vi "__READ_PM_1ch_E4419A.VI"(7 "GPIB":string="13") -> (3 "chA":dbl=-19.9032016 format="%.4f")   [LabVIEW 2017]
panel:
  # "TPD//133.40.220.247//2"
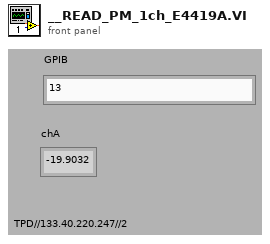
[diagram p1: front panel]
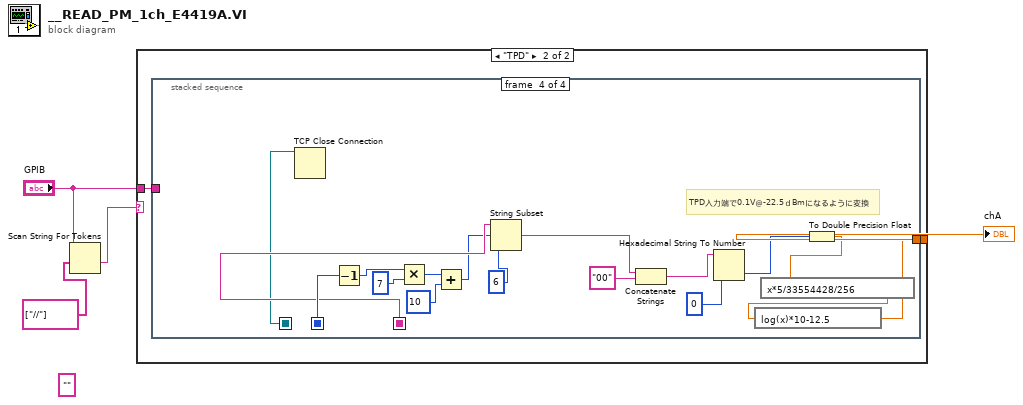
[diagram p0: block diagram]
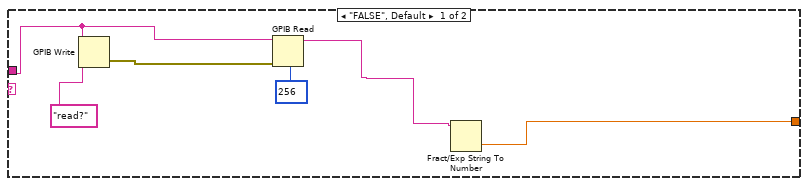
[diagram p2: hidden frame]
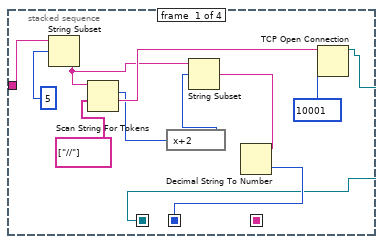
[diagram p3: hidden frame]
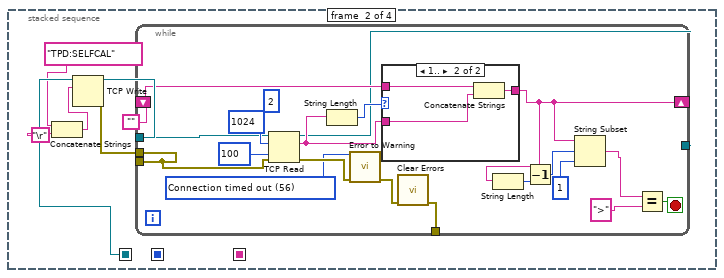
[diagram p4: hidden frame]
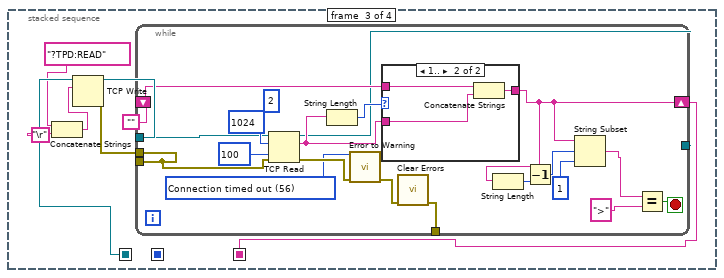
[diagram p6: hidden frame]
diagram:
  (unwired) ""
  n1 = Scan String For Tokens(7:string[] ["//"], 9:"GPIB") -> (1:w1:string)  [unwired: 4 in, 3 out]
  n2 = case shown="\"TPD\"" w1 {
    tunnel: [w10 w11] -> w4
    tunnel: "GPIB" -> [w5 w12]
    frame "FALSE", Default {
      n3 = GPIB Write(0:w5, 1:"read?") -> (6:w6:errorcluster)  [unwired: 3 in, 1 out]
      n4 = GPIB Read(0:w5, 1:256, 3:w6) -> (5:w9:string)  [unwired: 2 in, 2 out]
      n5 = Fract/Exp String To Number(string=w9) -> (number=w10:dbl)  [unwired: 3 in, 1 out]
    }
    frame "TPD" {
      n6 = stacked-sequence {
        seq-local: [w13 _ _ _] -> [_ w30 w61 w85]
        seq-local: [w14 _ _ _] -> [_ _ _ w101]
        seq-local: [_ _ w57 _] -> [_ _ _ w96]
        tunnel: w12 -> [w21 _ _ _]
        tunnel: [_ _ _ w86] -> w11
        frame #0 {
          n7 = String Subset(string=w21, offset (0)=5) -> (substring=w16:string)  [unwired: 1 in]
          n8 = Scan String For Tokens(7:string[] ["//"], 9:w16) -> (1:w20:string, 2:w19:i32)  [unwired: 4 in, 2 out]
          n9 = expression code="x+2"(w19) -> (w18:i32)
          n10 = String Subset(string=w16, offset (0)=w18) -> (substring=w17:string)  [unwired: 1 in]
          n11 = Decimal String To Number(string=w17) -> (number=w14:i32)  [unwired: 2 in, 1 out]
          n12 = TCP Open Connection(address=w20, remote port or service name=10001) -> (connection ID=w13:refnum<k5>)  [unwired: 3 in, 1 out]
        }
        frame #1 {
          n13 = Concatenate Strings("TPD:SELFCAL", "\r") -> (w24:string)
          n14 = TCP Write(connection ID=w30, data in=w24) -> (connection ID out=w28:refnum<k5>, error out=w27:errorcluster)  [unwired: 2 in, 1 out]
          n15 = while {
            tunnel: w28 -> [w48]
            shift-right: [w41] -> _
            shift-left: "" -> [w44]
            tunnel: [w31] -> _
            tunnel: [w34] -> _
            tunnel: [w32] -> _
            tunnel: w27 -> [w31]
            stop <- w36 stop-if-true
            (unwired) 2
            w46 = 56 items=["No Error", "Argument Error", "Memory Full", "Out of Zone", "End of File", "File Already Open", "Generic File IO Error", "File Not Found", "File Permission Error", "Disk Full", "Duplicate Path", "Too Many Files Open", "Not Enabled", "Resource File Not Found", "Cannot Add Resource", "Resource Not Found", "Image Not Found", "Image Memory Error", "Pen Does Not Exist", "Config Bad Type", "Config Token Not Found", "Config Parse Error", "Config Memory Error", "Bad External Code Format", "Bad External Code Offset", "External Code Not Present", "Null Window", "Destroy Window Mixup", "Null Menu", "Print Aborted", "Bad Print Record", "Print Driver Error", "Windows Error During Print", "Memory Error During Print", "Print Dialog Error", "Generic Print Error", "Invalid Device Refnum", "Device Not Found", "Device Parameter Error", "Device Unit Error", "Can't Open Device", "Device Call Aborted", "Generic Error", "Cancelled By User", "Object ID Too Low", "Object ID Too High", "Object Not In Heap", "Unknown Heap", "Bad DefProc ID", "DefProc Not In Table", "Message Out Of Range", "Null Method", "Unknown Message", "Manager Call Not Supported", "Bad address", "Connection In progress", "Connection timed out", "Connection is already in progress", "Network attribute not supported", "Network error", "Address in use", "System out of memory", "Connection aborted", "Connection refused", "Connection is not connected", "Connection is already connected", "Connection closed", "Initialize error (interapplication manager)", "Bad occurrence", "Wait on unbound occurrence handler", "Occurrence queue overflow", "Bad path", "Semaphore not signaled", "Unrecognized type (interapplication manager)"] ("1st Error to Convert")
            n16 = TCP Read(connection ID=w48, bytes to read=1024, error in (no error)=w31, 9:100) -> (connection ID out=w32:refnum<k5>, data out=w43:string, error out=w47:errorcluster)  [unwired: 1 in]
            n17 = String Length(string=w43) -> (length=w45:i32)
            n18 = call <vilib>:"Error to Warning.vi"("1st Error to Convert"=w46, "error in"=w47) -> ("warning out"=w35:errorcluster)  [unwired: 13 in]
            n19 = case shown="1.." w45 {
              tunnel: w43 -> [_ w51]
              tunnel: w44 -> [w50 w53]
              tunnel: [w50 w52] -> w41
              frame ..0 {
              }
              frame 1.. {
                n20 = Concatenate Strings(w53, w51) -> (w52:string)
              }
            }
            n21 = call <vilib>:"Clear Errors.vi"("error in (no error)"=w35) -> ("error out"=w34:errorcluster)  [unwired: 5 in, 1 out]
            n22 = String Length(string=w41) -> (length=w42:i32)
            n23 = Decrement(x=w42) -> (x-1=w40:i32)
            n24 = String Subset(string=w41, offset (0)=w40, length (rest)=1) -> (substring=w38:string)
            n25 = Equal?(x=w38, y=">") -> (x = y?=w36:bool)
          }
        }
        frame #2 {
          n26 = Concatenate Strings("?TPD:READ", "\r") -> (w54:string)
          n27 = TCP Write(connection ID=w61, data in=w54) -> (connection ID out=w59:refnum<k5>, error out=w58:errorcluster)  [unwired: 2 in, 1 out]
          n28 = while {
            tunnel: w59 -> [w79]
            shift-right: [w72] -> w57
            shift-left: "" -> [w75]
            tunnel: [w62] -> _
            tunnel: [w65] -> _
            tunnel: [w63] -> _
            tunnel: w58 -> [w62]
            stop <- w67 stop-if-true
            (unwired) 2
            w77 = 56 items=["No Error", "Argument Error", "Memory Full", "Out of Zone", "End of File", "File Already Open", "Generic File IO Error", "File Not Found", "File Permission Error", "Disk Full", "Duplicate Path", "Too Many Files Open", "Not Enabled", "Resource File Not Found", "Cannot Add Resource", "Resource Not Found", "Image Not Found", "Image Memory Error", "Pen Does Not Exist", "Config Bad Type", "Config Token Not Found", "Config Parse Error", "Config Memory Error", "Bad External Code Format", "Bad External Code Offset", "External Code Not Present", "Null Window", "Destroy Window Mixup", "Null Menu", "Print Aborted", "Bad Print Record", "Print Driver Error", "Windows Error During Print", "Memory Error During Print", "Print Dialog Error", "Generic Print Error", "Invalid Device Refnum", "Device Not Found", "Device Parameter Error", "Device Unit Error", "Can't Open Device", "Device Call Aborted", "Generic Error", "Cancelled By User", "Object ID Too Low", "Object ID Too High", "Object Not In Heap", "Unknown Heap", "Bad DefProc ID", "DefProc Not In Table", "Message Out Of Range", "Null Method", "Unknown Message", "Manager Call Not Supported", "Bad address", "Connection In progress", "Connection timed out", "Connection is already in progress", "Network attribute not supported", "Network error", "Address in use", "System out of memory", "Connection aborted", "Connection refused", "Connection is not connected", "Connection is already connected", "Connection closed", "Initialize error (interapplication manager)", "Bad occurrence", "Wait on unbound occurrence handler", "Occurrence queue overflow", "Bad path", "Semaphore not signaled", "Unrecognized type (interapplication manager)"] ("1st Error to Convert")
            n29 = TCP Read(connection ID=w79, bytes to read=1024, error in (no error)=w62, 9:100) -> (connection ID out=w63:refnum<k5>, data out=w74:string, error out=w78:errorcluster)  [unwired: 1 in]
            n30 = String Length(string=w74) -> (length=w76:i32)
            n31 = call <vilib>:"Error to Warning.vi"("1st Error to Convert"=w77, "error in"=w78) -> ("warning out"=w66:errorcluster)  [unwired: 13 in]
            n32 = case shown="1.." w76 {
              tunnel: w74 -> [_ w82]
              tunnel: w75 -> [w81 w84]
              tunnel: [w81 w83] -> w72
              frame ..0 {
              }
              frame 1.. {
                n33 = Concatenate Strings(w84, w82) -> (w83:string)
              }
            }
            n34 = call <vilib>:"Clear Errors.vi"("error in (no error)"=w66) -> ("error out"=w65:errorcluster)  [unwired: 5 in, 1 out]
            n35 = String Length(string=w72) -> (length=w73:i32)
            n36 = Decrement(x=w73) -> (x-1=w71:i32)
            n37 = String Subset(string=w72, offset (0)=w71, length (rest)=1) -> (substring=w69:string)
            n38 = Equal?(x=w69, y=">") -> (x = y?=w67:bool)
          }
        }
        frame #3 {
          # "TPD入力端で0.1V＠-22.5ｄBmになるように変換"
          n39 = TCP Close Connection(connection ID=w85) -> ()  [unwired: 2 in, 2 out]
          n40 = Decrement(x=w101) -> (x-1=w100:i32)
          n41 = Multiply(x=w100, y=7) -> (x*y=w98:i32)
          n42 = Add(x=w98, y=10) -> (x+y=w95:i32)
          n43 = String Subset(string=w96, offset (0)=w95, length (rest)=6) -> (substring=w93:string)
          n44 = Concatenate Strings(w93, "00") -> (w91:string)
          n45 = Hexadecimal String To Number(string=w91, default (0uL)=0) -> (number=w89:i32)  [unwired: 1 in, 1 out]
          n46 = To Double Precision Float(number=w89) -> (double precision float=w90:dbl)
          n47 = expression code="x*5/33554428/256"(w90) -> (w87:dbl)
          n48 = expression code="log(x)*10-12.5"(w87) -> (w86:dbl)
        }
      }
    }
  }
  "chA" <- w4
